vi "Configure Limit Test.vi"(5 "Lower Limit (0 V)":dbl, 6 "Upper Limit (0 V)":dbl, 7 "Fail Condition (0: Inside)":i32(ring) items=["Inside", "Outside"], 8 "error in (no error)":errorcluster, 9 "Source for Limit Test (0: Measurement1)":i32(ring) items=["Measurement1", "Measurement2", "Measurement3", "Measurement4", "Measurement5"], 10 "Enable Limit Test (F: Disable)":bool, 11 "VISA resource name":refnum<visa-resource-name>) -> (0 "error out":errorcluster, 3 "VISA resource name out":refnum<visa-resource-name>)   [LabVIEW 2020, in "Agilent 90000 Series.lvlib"]
doc: "Configures limit test parameters."
uses:
  Agilent 90000 Series.lvlib
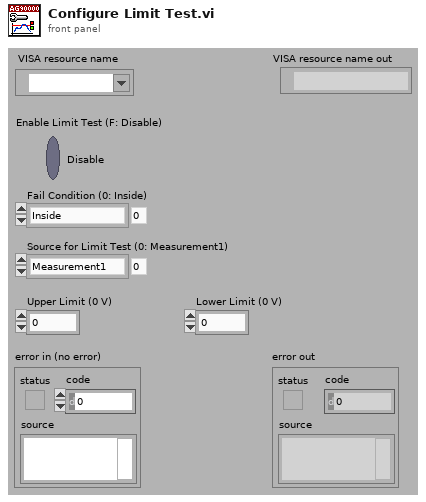
[diagram p1: front panel]
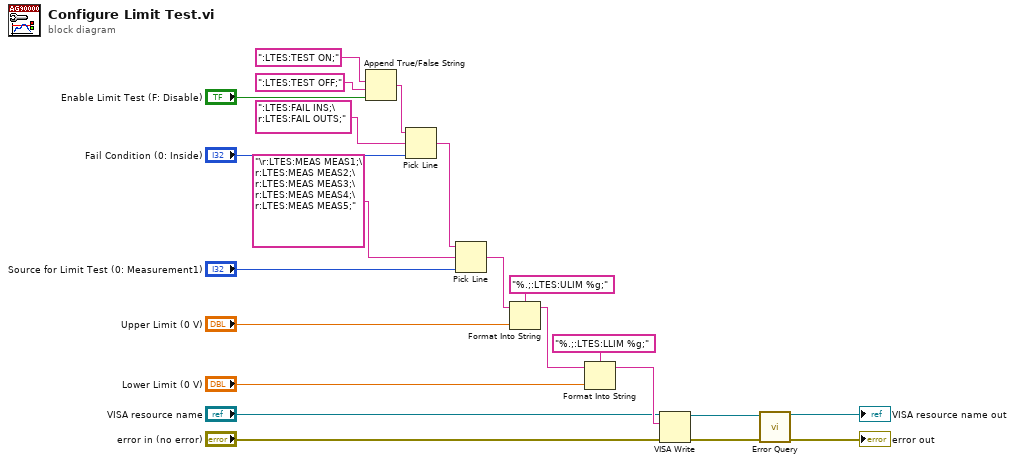
[diagram p0: block diagram]
diagram:
  n1 = Append True/False String(1:"Enable Limit Test (F: Disable)", 2:":LTES:TEST OFF;", 3:":LTES:TEST ON;") -> (0:w19:string)  [unwired: 1 out]
  n2 = Pick Line(string ("")=w19, multi-line string=":LTES:FAIL INS;\r:LTES:FAIL OUTS;", line index="Fail Condition (0: Inside)") -> (output string=w16:string)
  n3 = Pick Line(string ("")=w16, multi-line string="\r:LTES:MEAS MEAS1;\r:LTES:MEAS MEAS2;\r:LTES:MEAS MEAS3;\r:LTES:MEAS MEAS4;\r:LTES:MEAS MEAS5;", line index="Source for Limit Test (0: Measurement1)") -> (output string=w1:string)
  n4 = Format Into String(format string="%.;:LTES:ULIM %g;", initial string=w1, "Upper Limit (0 V)") -> (resulting string=w11:string)  [unwired: 1 in, 1 out]
  n5 = Format Into String(format string="%.;:LTES:LLIM %g;", initial string=w11, "Lower Limit (0 V)") -> (resulting string=w8:string)  [unwired: 1 in, 1 out]
  n6 = VISA Write(VISA resource name="VISA resource name", write buffer=w8, error in (no error)="error in (no error)") -> (VISA resource name out=w5:refnum<visa-resource-name>, error out=w4:errorcluster)  [unwired: 1 out]
  n7 = call "Error Query.vi"("error in (no error)"=w4, "VISA resource name"=w5) -> ("error out"=→"error out":errorcluster, "VISA resource name out"=→"VISA resource name out":refnum<visa-resource-name>)  [unwired: 8 out]
